vi "New.vi"(7 "Nailed?":bool, 8 "error in":errorcluster, 9 "Voltage":dbl, 10 "Number of Coconuts":i32, 11 "Type of Parrot":enum16{"European", "African", "Norwegian Blue"}(ring)) -> (0 "error out":errorcluster, 3 "Parrot out":refnum<class "Parrot.lvclass">)   [LabVIEW 2020, in "Parrot.lvclass"]
uses:
  Parrot.lvclass
  Parrot.lvclass/Parrot.ctl
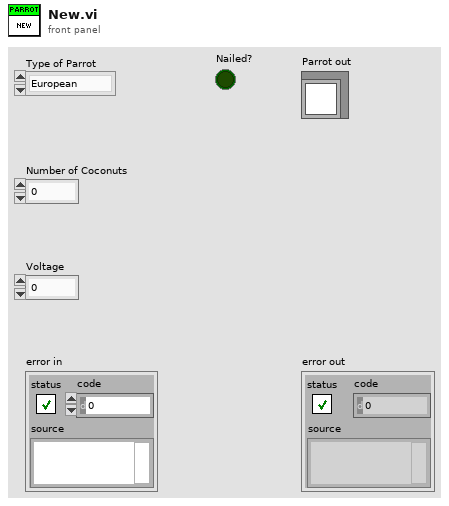
[diagram p1: front panel]
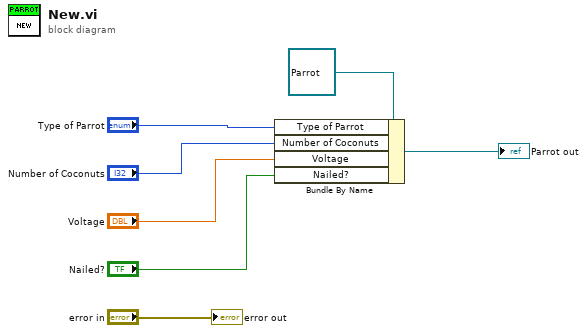
[diagram p0: block diagram]
diagram:
  n1 = Bundle By Name(cluster=refnum<class "Parrot.lvclass"> refnum ("Parrot out"), "Type of Parrot"="Type of Parrot", "Number of Coconuts"="Number of Coconuts", "Voltage"="Voltage", "Nailed?"="Nailed?") -> (→"Parrot out":refnum<class "Parrot.lvclass">)
  "error out" <- "error in"
